vi "Set Slave Info.vi"(6 "Distributed Clock (F)":bool, 7 "Prepend":bool, 8 "error in (no error)":errorcluster, 9 "Slave #":u16, 10 "Slave Name":string, 11 "Item Ref in":T1 format="%.0x") -> (0 "error out":errorcluster, 3 "Item Ref out":T1 format="%.0x")   [LabVIEW 2020, in "SEECD System Explorer.lvlib"]
uses:
  SEECD System Explorer.lvlib
  <vilib>/NI VeriStand/Custom Device API/Custom Device API.lvlib
  Shared/Globals/Property Strings.vi
  Shared/SEECD Shared.lvlib
  <vilib>/NI VeriStand/Custom Device API/Set Item Property (Boolean).vi
  <vilib>/NI VeriStand/Custom Device API/Set Item Property (U16).vi
  <vilib>/NI VeriStand/Custom Device API/Custom Device Item Ref.ctl
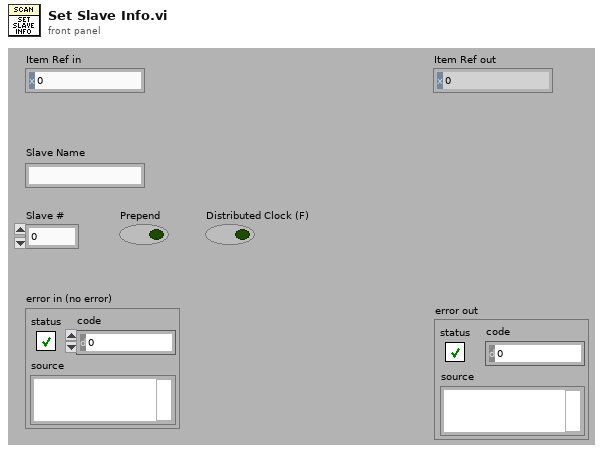
[diagram p1: front panel]
types:
  T1 = typedef "Custom Device API.lvlib/Custom Device Item Ref.ctl" = u64
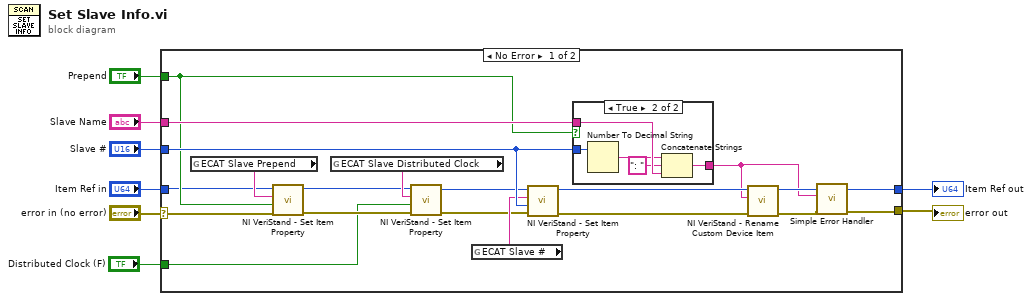
[diagram p0: block diagram]
diagram:
  n1 = case shown="No Error" "error in (no error)" {
    selector: "error in (no error)" -> [w19 w34]
    tunnel: "Item Ref in" -> [w20 w35]
    tunnel: "Slave Name" -> [w27 _]
    tunnel: "Slave #" -> [w26 _]
    tunnel: [w10 w34] -> w4
    tunnel: [w18 w35] -> w3
    tunnel: "Prepend" -> [w22 _]
    tunnel: "Distributed Clock (F)" -> [w13 _]
    frame No Error {
      n2 = global read "Property Strings.vi" "ECAT Slave Prepend"() -> (w21:string)
      n3 = call-poly <vilib>:"NI VeriStand - Set Item Property.vi"("error in (no error)"=w19, "Value"=w22, "Property Name"=w21, "Item Ref in"=w20) -> ("error out"=w17:errorcluster, "Item Ref out"=w14:T1)  [unwired: 5 in, 1 out]
      n4 = global read "Property Strings.vi" "ECAT Slave Distributed Clock"() -> (w15:string)
      n5 = call-poly <vilib>:"NI VeriStand - Set Item Property.vi"("error in (no error)"=w17, "Value"=w13, "Property Name"=w15, "Item Ref in"=w14) -> ("error out"=w16:errorcluster, "Item Ref out"=w12:T1)  [unwired: 5 in, 1 out]
      n6 = global read "Property Strings.vi" "ECAT Slave #"() -> (w23:string)
      n7 = call-poly <vilib>:"NI VeriStand - Set Item Property.vi"("error in (no error)"=w16, "Value"=w26, "Property Name"=w23, "Item Ref in"=w12) -> ("error out"=w25:errorcluster, "Item Ref out"=w24:T1)  [unwired: 5 in, 1 out]
      n8 = case shown="True" w22 {
        tunnel: [w28 w33] -> w9
        tunnel: w27 -> [w28 w32]
        tunnel: w26 -> [_ w31]
        frame False {
        }
        frame True {
          n9 = Number To Decimal String(number=w31) -> (decimal integer string=w30:string)  [unwired: 1 in]
          n10 = Concatenate Strings(w30, ": " ("string"), w32) -> (w33:string)
        }
      }
      n11 = call <vilib>:"NI VeriStand - Rename Custom Device Item.vi"("error in (no error)"=w25, "New Name"=w9, "Item Ref in"=w24) -> ("error out"=w11:errorcluster, "Item Ref out"=w18:T1)  [unwired: 1 in, 6 out]
      n12 = call <vilib>:"Simple Error Handler.vi"("error source (\" \")"=w9, "error in (no error)"=w11) -> ("error out"=w10:errorcluster)  [unwired: 1 in, 6 out]
    }
    frame Error {
    }
  }
  "error out" <- w4
  "Item Ref out" <- w3
